vi "PID measuring automatic VI.vi"() -> ()   [LabVIEW 2025]
uses:
  <vilib>/addons/control/pid/pid.llb/PID Advanced (DBL).vi
  <vilib>/addons/control/pid/NI_PID_pid.lvlib
panel:
  out "LCV":dbl(knob) scale=0.0..100.0 scale format="%#_3g"
  in  "stop":bool
  out "Waveform Chart":T1(graph)
  out "PV output":dbl(slide) scale=0.0..100.0
  in  "process parameters":T2={"static gain"=2.5, "lag (s)"=2.5, "deadtime (s)"=0.001, "load"=0.0, "deadband"=0.0, "sensor noise"=0.0, "initial PV"=30.0, "plant noise"=0.0} {"plant noise" format="%.2f"; "initial PV" format="%.2f"; "sensor noise" format="%.2f"; "lag (s)" format="%.2f"; "deadtime (s)" format="%.2f"; "deadband" format="%.1f"; "load" format="%.2f"; "static gain" format="%.2f"}
  in  "set point(SP)":dbl(slide) scale=0.0..100.0
  in  "PID gains":T3={"proportional gain (Kc)"=1.0, "integral time (Ti, min)"=0.01, "derivative time (Td, min)"=0.0} {"derivative time (Td, min)" format="%.3f"; "integral time (Ti, min)" format="%.3f"; "proportional gain (Kc)" format="%.3f"}
  in  "output range":cluster{"output high":dbl, "output low":dbl}={"output high"=100.0, "output low"=-100.0} {"output low" format="%.2f"; "output high" format="%.2f"}
  in  "auto? (T)":bool=TRUE
  in  "Liquid contriol":dbl format="%.2f"
  # "PID"
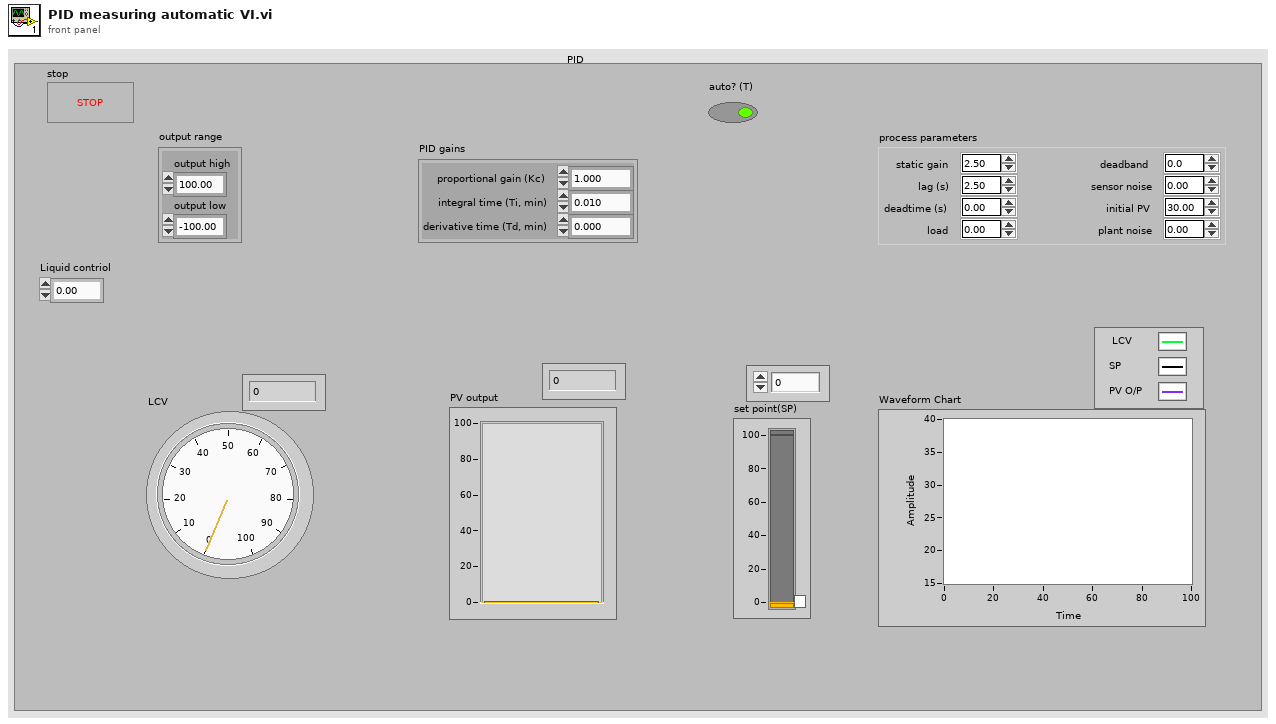
[diagram p1: front panel]
types:
  T1 = cluster{"Liquid contriol":dbl, "set point(SP) ":dbl, "Plant Output":dbl}
  T2 = cluster{"static gain":dbl, "lag (s)":dbl, "deadtime (s)":dbl, "load":dbl, "deadband":dbl, "sensor noise":dbl, "initial PV":dbl, "plant noise":dbl}
  T3 = cluster{"proportional gain (Kc)":dbl, "integral time (Ti, min)":dbl, "derivative time (Td, min)":dbl}
  T4 = cluster{"output":dbl, "set point(SP) ":dbl, "Plant Output":dbl}
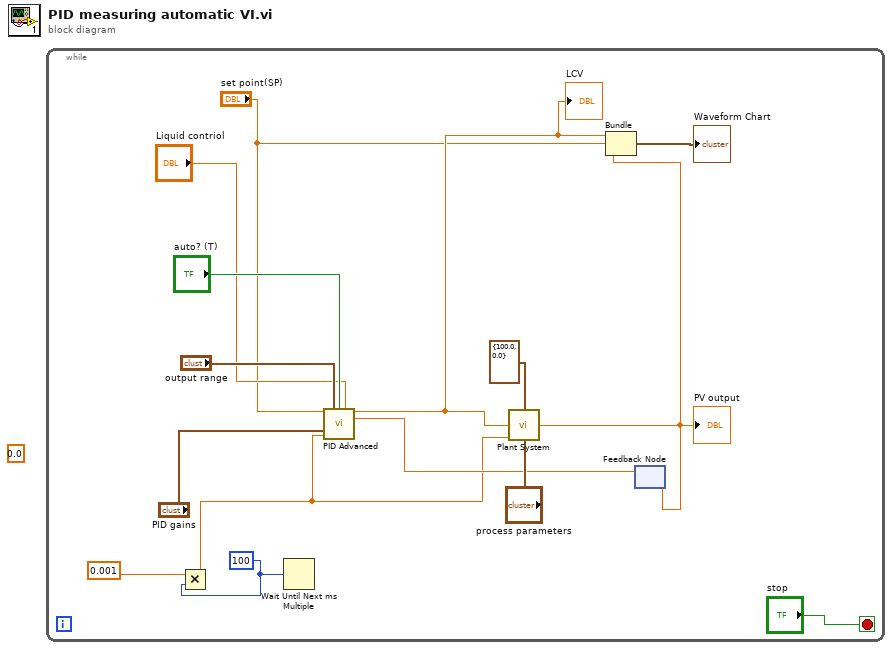
[diagram p0: block diagram]
diagram:
  (unwired) 0.0 ("Plant Output")
  n1 = while {
    stop <- "stop" stop-if-true
    w2 = u32 100 ("millisecond multiple")
    n2 = Multiply(x=0.001, y=w2) -> (x*y=w1:dbl)
    n3 = Wait Until Next ms Multiple(millisecond multiple=w2) -> ()  [unwired: 1 out]
    n4 = feedback #1() -> (w10:dbl)  [unwired: 1 in]
    n5 = call-poly <vilib>:"PID Advanced.vi"("setpoint"="set point(SP)", "output range"="output range", "auto? (T)"="auto? (T)", "manual control"="Liquid contriol", "process variable"=w10, "PID gains"="PID gains", "dt (s)"=w1) -> ("output"=w4:dbl)  [unwired: 7 in, 1 out]
    "LCV" <- w4
    n6 = call "Plant System.vi"("output saturation range"=cluster{"output high":dbl, "output low":dbl} {"output high"=100.0, "output low"=0.0}, "Plant Input"=w4, "dt (s)"=w1, "process parameters"="process parameters") -> ("Plant Output"=w8:dbl)  [unwired: 11 in]
    "PV output" <- w8
    n7 = Bundle("output"=w4, "set point(SP)"="set point(SP)", "Plant Output"=w8) -> (→"Waveform Chart":T4)  [unwired: 1 in]
    n8 = feedback-in #1(w8) -> ()
  }
